vi "SetScrollBarVisibility.vi"(9 "Array Vertical Scrollbar Visibility":T2(array[ring]), 10 "Array HorizScrollBarViz":T2(array[ring]), 11 "Panes":T1) -> ()   [LabVIEW 2022 SP3, in "PentaPanesLibrary.lvlib" / "PentaPanes.lvclass"]
uses:
  PentaPanes.lvclass
  PanesCluster.ctl
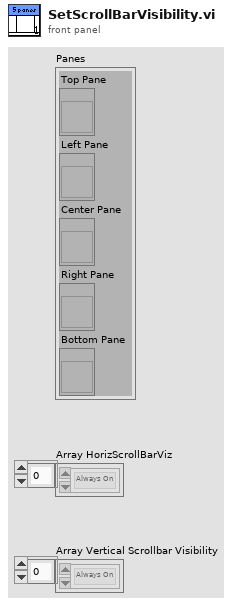
[diagram p1: front panel]
types:
  T1 = typedef "PentaPanesLibrary.lvlib/PentaPanes.lvclass/PanesCluster.ctl" = cluster{"Top Pane":refnum<vi>, "Left Pane":refnum<vi>, "Center Pane":refnum<vi>, "Right Pane":refnum<vi>, "Bottom Pane":refnum<vi>}
  T2 = enum16{"Always On", "Always Off", "Off While Running"}[]
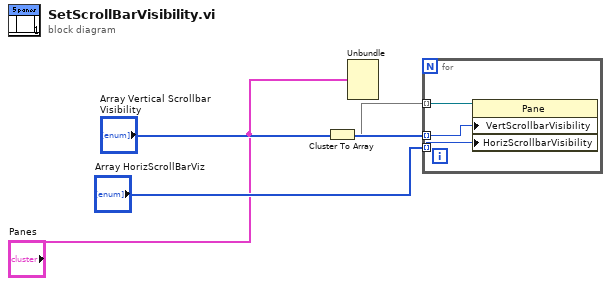
[diagram p0: block diagram]
diagram:
  n1 = Cluster To Array(cluster="Panes") -> (array=w2:refnum<vi>[])
  n2 = Unbundle("Panes") -> ()  [unwired: 5 out]
  n3 = for {
    tunnel: w2 -> [w7] mode=indexing
    tunnel: "Array Vertical Scrollbar Visibility" -> [w6] mode=indexing
    tunnel: "Array HorizScrollBarViz" -> [w5] mode=indexing
    n4 = property class="Pane"(reference=w7, "VertScrollbarVisibility"=w6, "HorizScrollbarVisibility"=w5) -> ()  [unwired: 1 in, 2 out]
  }
